vi "TEST_ASIC_SUM_NEW.vi"(7 "Serial Number":string="SN_143t", 8 "error in (no error)":errorcluster, 11 "Instrument VISA in":T1={"AWG VISA"="AgilentGenerator1", "Oscilloscope  VISA "="AgilentOsciloscope", "Integration Board IP"="172.16.17.47", "connection ID"=refnum, "report out"=refnum, "report file path"=path "C:/Users/omartinez/Desktop/L0nL1_Results"}) -> (0 "error out":errorcluster, 3 "Instrument VISA out 2":T1={"AWG VISA"="AgilentGenerator1", "Oscilloscope  VISA "="AgilentOsciloscope", "Integration Board IP"="172.16.17.47", "connection ID"=refnum, "report out"=refnum, "report file path"=path "C:/Users/omartinez/Desktop/L0nL1_Results"})   [LabVIEW 2012]
uses:
  <vilib>/Utility/NIReport.llb/NI_report.lvclass
  <vilib>/Utility/NIReport.llb/HTML/NI_HTML.lvclass
  <instrlib>/Agilent 8000 Series/Public/Configure/Configure Math (Binary Operation).vi
  Sum_Abrilader/L0_Sum_Adder Folder/C/Program Files/National Instruments/LabVIEW 2012/instr.lib/Agilent 8000 Series/Public/Data/Low Level/Fetch Measurement (More).vi
  <instrlib>/Agilent 8000 Series/Agilent 8000 Series.lvlib
  Sum_Abrilader/L0_Sum_Adder Folder/C/Program Files/National Instruments/LabVIEW 2012/instr.lib/Agilent 81150/Agilent 81150.lvlib
panel:
  in  "Amp Scaler":dbl=2.0
  in  "IB_Clip":i32[](array[numeric])=[7, 23, 31, 63]
  in  "Channels":i32[](array[numeric])=[0, 1, 2, 3, 4, 5, 6]
  in  "Voltages":dbl[](array[numeric])=[0.05, 0.1, 0.2, 0.5, 0.8]
  in  "Atenuation":i32[](array[numeric])=[0, 15]
  in  "Clip Select":i32[](array[numeric])=[1, 2, 3]
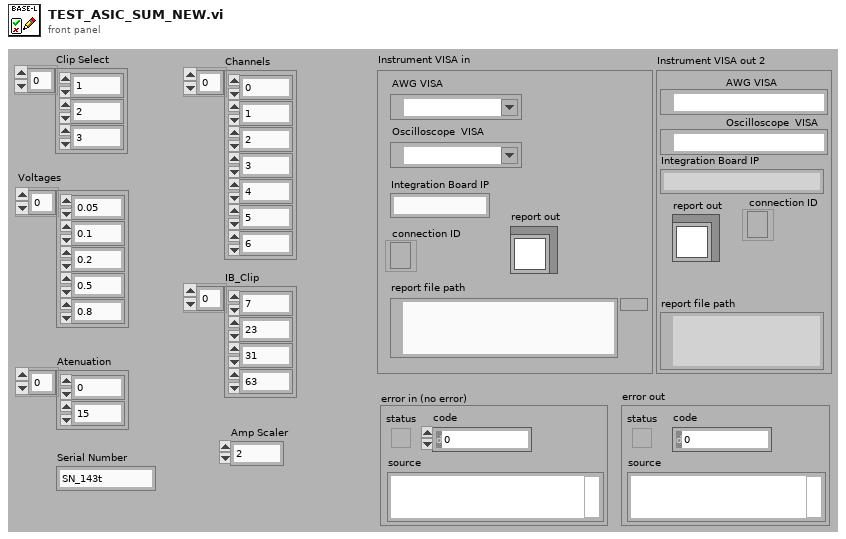
[diagram p1: front panel]
types:
  T1 = cluster{"AWG VISA":refnum<visa-resource-name>, "Oscilloscope  VISA ":refnum<visa-resource-name>, "Integration Board IP":string, "connection ID":refnum<k5>, "report out":refnum<class "NI_report.lvclass">, "report file path":path}
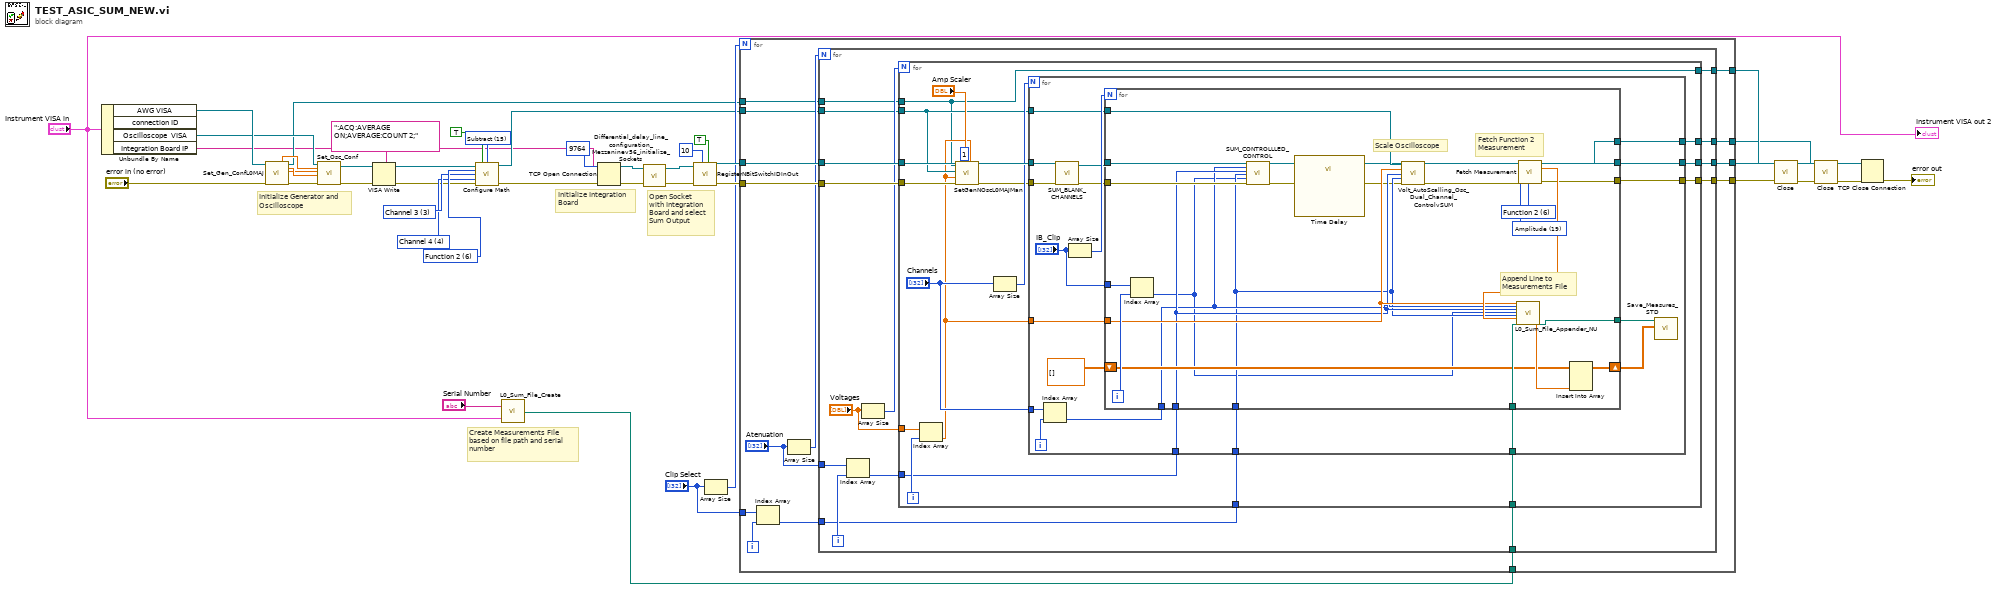
[diagram p0: block diagram]
diagram:
  w29 = u16 6 items=["Function 1"=5, "Function 2"=6, "Function 3"=7, "Function 4"=8] ("Math Channel (5: Function 1)")
  w30 = u16 15 items=["Add"=12, "Divide"=13, "Multiply"=14, "Subtract"=15, "Common Mode"=16, "Versus"=17] ("Math Operation (12: Add)")
  w28 = 3 items=["Channel 1"=1, "Channel 2"=2, "Channel 3"=3, "Channel 4"=4] ("Channel (1: Channel 1)")
  w27 = 4 items=["Channel 1"=1, "Channel 2"=2, "Channel 3"=3, "Channel 4"=4] ("Channel (1: Channel 1)")
  # "Open Socket\nwith Integration\nBoard and select\nSum Output"
  # "Initialize Integration\nBoard"
  # "Create Measurements File\nbased on file path and serial\nnumber"
  # "Initialize Generator and \nOscilloscope"
  n1 = Unbundle By Name("Instrument VISA in") -> ("AWG VISA"=w26:refnum<visa-resource-name>, "Oscilloscope  VISA"=w25:refnum<visa-resource-name>, "Integration Board IP"=w6:string)  [unwired: 1 out]
  n2 = call "Set_Gen_ConfL0MAJ.vi"("AWG VISA"=w26, "error in (no error)"="error in (no error)") -> ("Amplitude 1 OUT"=w34:dbl, "VISA resource name out"=w21:refnum<visa-resource-name>, "Pulse Width in seconds 1 OUT"=w33:dbl, "Trigger Level 1"=w32:dbl, "error out"=w35:errorcluster)  [unwired: 10 in, 3 out]
  n3 = call "Set_Osc_Conf.vi"("VISA resource name"=w25, "Amplitude IN"=w34, "Trigger Level IN"=w32, "Pulse Width in seconds IN"=w33, "error in (no error)"=w35) -> ("VISA resource name out"=w13:refnum<visa-resource-name>, "error out"=w16:errorcluster)  [unwired: 13 in]
  n4 = VISA Write(VISA resource name=w13, write buffer=":ACQ:AVERAGE ON;AVERAGE:COUNT 2;", error in (no error)=w16) -> (VISA resource name out=w12:refnum<visa-resource-name>, error out=w15:errorcluster)  [unwired: 1 out]
  n5 = call-poly <instrlib>:"Configure Math.vi"("VISA resource name"=w12, "Enable Math Channel (T:Enable)"=TRUE, "Math Operation (12: Add)"=w30, "Math Channel (5: Function 1)"=w29, "Math Operand (1: Channel 1)"=w28, "Math Operand (2: Channel 2)"=w27, "error in (no error)"=w15) -> ("VISA resource name out"=w20:refnum<visa-resource-name>, "error out"=w5:errorcluster)  [unwired: 7 in]
  n6 = call "L0_Sum_File_Create.vi"("input cluster"="Instrument VISA in", "Serial Number"="Serial Number") -> ("appended path"=w18:path)
  n7 = TCP Open Connection(address=w6, remote port or service name=9764, error in (no error)=w5) -> (connection ID=w4:refnum<k5>, error out=w3:errorcluster)  [unwired: 2 in]
  n8 = call "Differential_delay_line_configuration_Mezzaninev56_initialize_Sockets.vi"("connection ID"=w4, "error in (no error)"=w3) -> ("connection ID out"=w1:refnum<k5>, "error out 2"=w2:errorcluster)  [unwired: 6 in]
  n9 = call "RegisterNBitSwitchIDInOut.vi"("Switch Bit"=TRUE, "N Bit"=10, "error in (no error)"=w2, "connection ID"=w1) -> ("error out"=w39:errorcluster, "connection ID out"=w38:refnum<k5>)  [unwired: 5 in]
  n10 = Array Size(array="Clip Select") -> (size(s)=w23:i32)
  n11 = for {
    N: w23 -> [_]
    tunnel: [w56] -> w9
    tunnel: [w55] -> w40
    tunnel: w39 -> [w54]
    tunnel: w38 -> [w53]
    tunnel: "Clip Select" -> [w51]
    tunnel: w21 -> [w48]
    tunnel: w20 -> [w47]
    tunnel: w18 -> [w45]
    tunnel: [w44] -> w8
    tunnel: [w43] -> w7
    i -> [w52]
    n12 = Index Array(array=w51, index=w52) -> (element=w46:i32)
    n13 = Array Size(array="Atenuation") -> (size(s)=w49:i32)
    n14 = for {
      N: w49 -> [_]
      tunnel: [w71] -> w56
      tunnel: [w70] -> w55
      tunnel: w54 -> [w69]
      tunnel: w53 -> [w68]
      tunnel: "Atenuation" -> [w66]
      tunnel: w48 -> [w63]
      tunnel: w47 -> [w62]
      tunnel: w46 -> [w60]
      tunnel: w45 -> [w59]
      tunnel: [w58] -> w44
      tunnel: [w57] -> w43
      i -> [w67]
      n15 = Index Array(array=w66, index=w67) -> (element=w61:i32)
      n16 = Array Size(array="Voltages") -> (size(s)=w64:i32)
      n17 = for {
        N: w64 -> [_]
        tunnel: [w89] -> w71
        tunnel: [w88] -> w70
        tunnel: w69 -> [w80]
        tunnel: w68 -> [w87]
        tunnel: "Voltages" -> [w85]
        tunnel: w63 -> [w73]
        tunnel: w62 -> [w76]
        tunnel: w61 -> [w78]
        tunnel: w60 -> [w77]
        tunnel: w59 -> [w74]
        tunnel: [w73] -> w58
        tunnel: [w72] -> w57
        i -> [w86]
        n18 = Index Array(array=w85, index=w86) -> (element=w75:dbl)
        n19 = call "SetGenNOscL0MAJMan.vi"("Input Voltage"=w75, "Amp Scaler"="Amp Scaler", "NChannels"=1, "error in (no error)"=w80, "Output Voltage"=w75, "VISA resource name"=w76, "AWG VISA"=w73) -> ("error out 2"=w79:errorcluster)  [unwired: 4 in]
        n20 = Array Size(array="Channels") -> (size(s)=w83:i32)
        n21 = for {
          N: w83 -> [_]
          tunnel: [w109] -> w89
          tunnel: [w108] -> w88
          tunnel: w79 -> [w107]
          tunnel: w87 -> [w91]
          tunnel: "Channels" -> [w105]
          tunnel: w78 -> [w101]
          tunnel: w77 -> [w100]
          tunnel: w76 -> [w99]
          tunnel: w75 -> [w98]
          tunnel: w74 -> [w97]
          tunnel: [w93] -> w72
          i -> [w106]
          n22 = Index Array(array=w105, index=w106) -> (element=w102:i32)
          n23 = call "SUM_BLANK_CHANNELS.vi"("error in"=w107, "connection ID in"=w91) -> ("error out"=w92:errorcluster, "connection ID out"=w90:refnum<k5>)  [unwired: 8 in]
          n24 = Array Size(array="IB_Clip") -> (size(s)=w103:i32)
          n25 = for {
            N: w103 -> [_]
            tunnel: [w127] -> w109
            tunnel: [w117] -> w108
            tunnel: w92 -> [w120]
            tunnel: w90 -> [w118]
            tunnel: "IB_Clip" -> [w133]
            tunnel: w102 -> [w115]
            tunnel: w101 -> [w116]
            tunnel: w100 -> [w114]
            tunnel: w99 -> [w126]
            tunnel: w98 -> [w125]
            tunnel: w97 -> [w124]
            tunnel: [w123] -> w96
            shift-right: [w121] -> w94
            shift-left: dbl[][] [] ("Y") -> [w122]
            tunnel: [w110] -> w93
            i -> [w134]
            w132 = 19 items=["Rise Time", "Fall Time", "Frequency", "Period", "Voltage RMS(AC)", "Voltage RMS(DC)", "Voltage RMS (AC,cycle)", "Voltage RMS (DC,cycle)", "Voltage Max", "Voltage Min", "Voltage Middle", "Voltage Vpp", "Voltage High", "Voltage Low", "Voltage Average", "Voltage Average (cycle)", "Width Negative", "Width Positive", "Duty Cycle Positive", "Amplitude", "Overshoot", "Preshoot", "Voltage Base", "Voltage Upper", "Time Max", "Time Min", "Color Grade Crossing", "Color Grade Eye Width", "Color Grade Eye Height", "Color Grade Eye Q-Factory", "Color Grade Eye Duty Cycle Distortion(Percent)", "Color Grade Eye Duty Cycle Distortion(Time)", "Color Grade Eye Jitter(PP)", "Color Grade Eye Width(RMS)", "Cycle-cycle Duty Jitter(Rising)", "Cycle-cycle Duty Jitter(Falling)", "Cycle-cycle Jitter(Rising)", "Cycle-cycle Jitter(Falling)", "Cycle-cycle - Width", "Cycle-cycle + Width", "Date Rate", "Unit Interval", "FFT Delta Frequency", "FFT Delta Magnitude", "FFT Frequency", "FFT Magnitude", "Slew Rate", "Area (Entire Display)", "Area(Single Cycle)", "Duty Cycle (Rising)", "Duty Cycle (Falling)"] ("Measurement Function (0: Rise Time)")
            w131 = 6 items=["Channel 1"=1, "Channel 2"=2, "Channel 3"=3, "Channel 4"=4, "Function 1"=5, "Function 2"=6, "Function 3"=7, "Function 4"=8, "Memory 1"=9, "Memory 2"=10, "Memory 3"=11, "Memory 4"=12] ("Channel (1: Channel 1)")
            # "Scale Oscilloscope"
            # "Append Line to \nMeasurements File"
            # "Fetch Function 2\nMeasurement"
            n26 = Index Array(array=w133, index=w134) -> (element=w113:i32)
            n27 = call "SUM_CONTROLLLED_CONTROL.vi"("connection ID in"=w118, "Channel Enable"=w115, "Attenuation Select"=w116, "Clipping Select"=w114, "Ib Clip select"=w113, "error in"=w120) -> ("connection ID out"=w117:refnum<k5>, "error out"=w119:errorcluster)  [unwired: 12 in]
            n28 = call "Time Delay"("error in (no error)"=w119) -> ("error out"=w112:errorcluster)  [unwired: 10 in]
            n29 = call "Volt_AutoScalling_Osc_Dual_Channel_ControlvSUM.vi"("VISA Oscilloscope"=w126, "Voltage In"=w125, "Att"=w116, "Clip"=w114, "error in"=w112) -> ("VISA resource name out"=w111:refnum<visa-resource-name>, "error out"=w129:errorcluster)  [unwired: 9 in]
            n30 = call-poly "Fetch Measurement.vi"("VISA resource name"=w111, "Channel (1: Channel 1)"=w131, "Measurement Function (0: Rise Time)"=w132, "error in (no error)"=w129) -> ("VISA resource name out"=w110:refnum<visa-resource-name>, "Measurement"=w130:dbl, "error out"=w127:errorcluster)  [unwired: 9 in]
            n31 = call "L0_Sum_File_Appender_NU.vi"("Vin"=w125, "CH"=w115, "Att"=w116, "IbClip"=w113, "Clip"=w114, "Vmeas"=w130, "file path (dialog if empty)"=w124) -> ("appended array"=w128:dbl[], "file path (dialog if empty) 2"=w123:path)  [unwired: 19 in]
            n32 = Insert Into Array(array=w122, new element=w128) -> (w121:dbl[][])  [unwired: 2 in]
          }
          n33 = call "Save_Measures_STD.vi"("Data in"=w94, "file path (dialog if empty)"=w96) -> ()  [unwired: 10 in]
        }
      }
    }
  }
  n34 = call <instrlib>:"Close.vi"("error in (no error)"=w9, "VISA resource name"=w8) -> ("error out"=w11:errorcluster)  [unwired: 9 in]
  n35 = call <instrlib>:"Close.vi"("error in (no error)"=w11, "VISA resource name"=w7) -> ("error out"=w10:errorcluster)  [unwired: 9 in]
  n36 = TCP Close Connection(connection ID=w40, error in (no error)=w10) -> (error out=→"error out":errorcluster)  [unwired: 1 in, 1 out]
  "Instrument VISA out 2" <- "Instrument VISA in"
